vi "CC Check Pressure Alarms.vi"(8 "error in (no error)":errorcluster, 9 "Enabled?":bool[](array[boolean]), 10 "Pressure Alarm Level":dbl format="%^_3g", 11 "Presssure Data":dbl[](array[numeric])) -> (0 "error out":errorcluster, 2 "Alarms":T1[](array[typedef]), 3 "Alarm":bool)   [LabVIEW 2024]
uses:
  typedefs/CC cluster Alarm Data.ctl
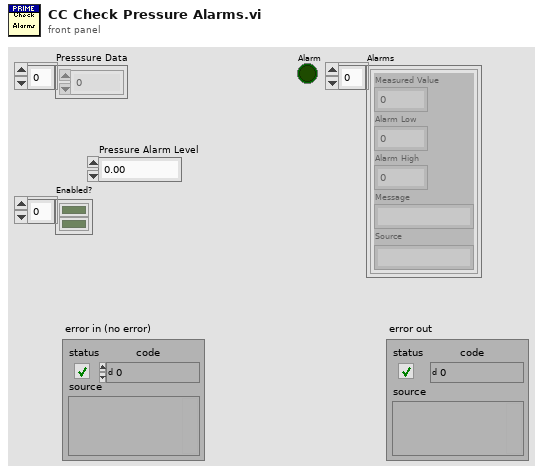
[diagram p1: front panel]
types:
  T1 = typedef "CC cluster Alarm Data.ctl" = cluster{"Measured Value":dbl, "Alarm Low":dbl, "Alarm High":dbl, "Message":string, "Source":string}
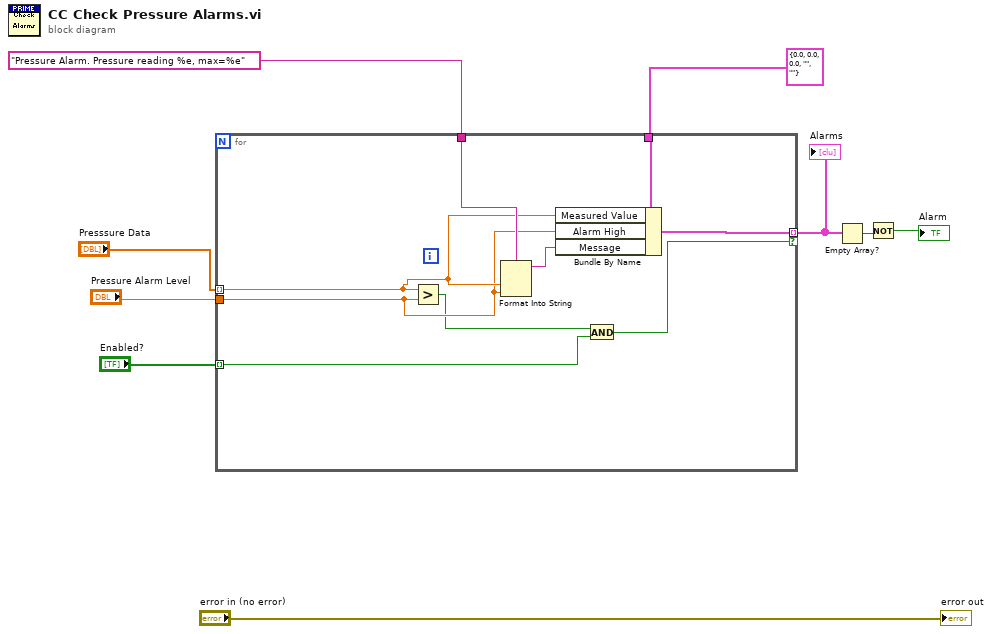
[diagram p0: block diagram]
diagram:
  n1 = for {
    tunnel: "Pressure Alarm. Pressure reading %e, max=%e" ("format string") -> [w18]
    tunnel: "Presssure Data" -> [w15] mode=indexing
    tunnel: "Pressure Alarm Level" -> [w14]
    tunnel: T1 {"Measured Value"=0.0, "Alarm Low"=0.0, "Alarm High"=0.0, "Message"="", "Source"=""} -> [w17]
    tunnel: [w16] -> w4 mode=indexing if=w13
    tunnel: "Enabled?" -> [w12] mode=indexing
    n2 = Greater?(x=w15, y=w14) -> (0:w10:bool)
    n3 = Format Into String(format string=w18, w15, w14) -> (resulting string=w11:string)  [unwired: 2 in, 1 out]
    n4 = Bundle By Name(cluster=w17, "Measured Value"=w15, "Alarm High"=w14, "Message"=w11) -> (w16:T1)
    n5 = And(x=w10, y=w12) -> (x .and. y?=w13:bool)
  }
  "Alarms" <- w4
  n6 = Empty Array?(array=w4) -> (empty?=w3:bool)
  n7 = Not(x=w3) -> (.not. x?=→"Alarm":bool)
  "error out" <- "error in (no error)"
